vi "Configure.vi"(8 "error in (no error)":errorcluster, 11 "configuration in":refnum<class "configurable.lvclass">) -> (0 "error out":errorcluster, 3 "configuration out":refnum<class "configurable.lvclass">)   [LabVIEW 2020, in "eos.lvlib" / "configurable.lvclass"]
uses:
  configurable.lvclass
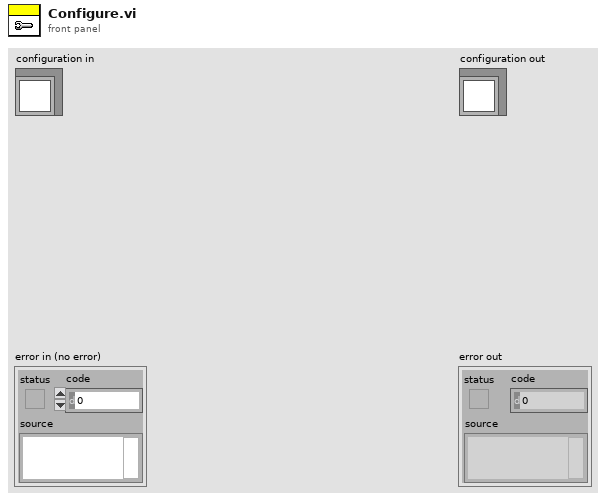
[diagram p1: front panel]
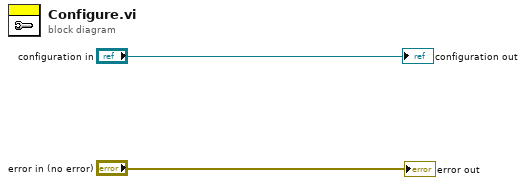
[diagram p0: block diagram]
diagram:
  "error out" <- "error in (no error)"
  "configuration out" <- "configuration in"
